vi "Test device info.vi"() -> ()   [LabVIEW 2020, in "XML Handler.lvclass"]
uses:
  XML Handler.lvclass
  Devices/Controls/Device Information Cluster.ctl
  Devices/Controls/Register to Write.ctl
  XML Handler.lvclass/XML Handler.ctl
  <resource>/objmgr/DOMUserDefRef.rc
  Test Framework/Test Framework.lvclass
  Devices/PIC-device/PIC-Device.lvclass
  Devices/Device.lvclass
panel:
  in  "Output File Folder":path
  out "XML":string
  in  "Device Information":T1[](array[typedef])
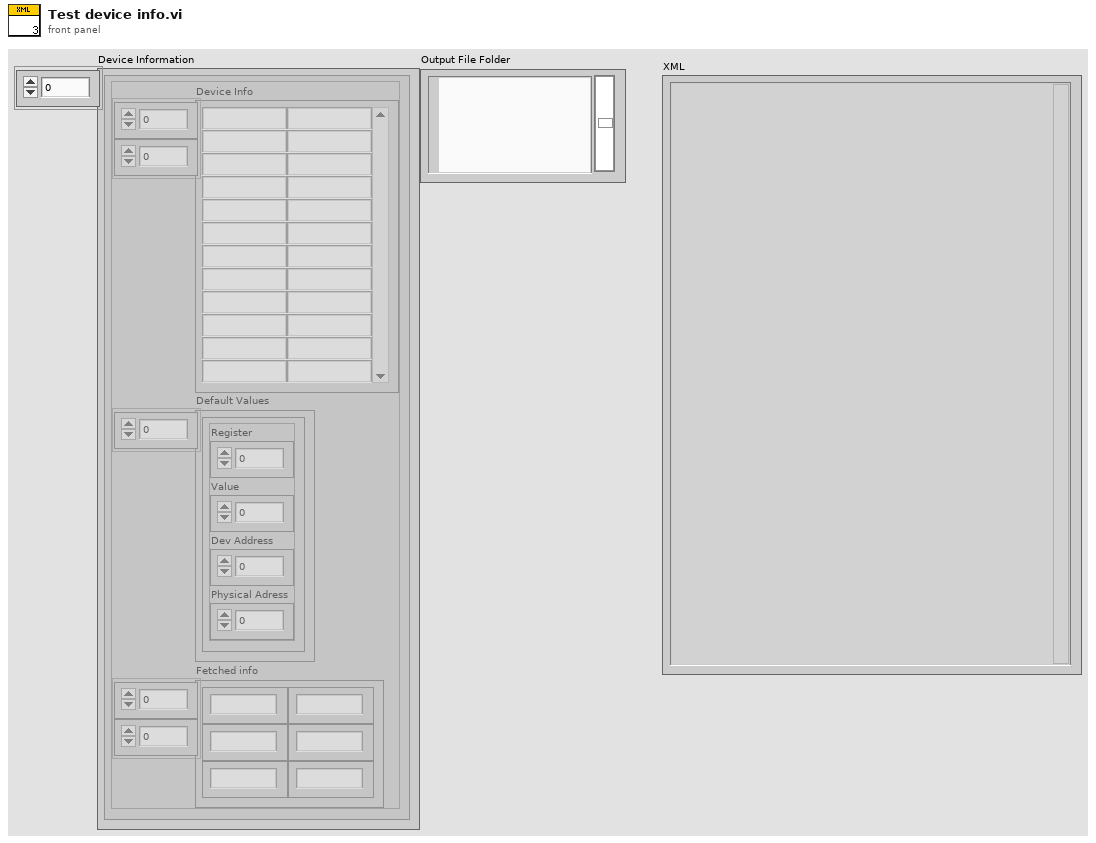
[diagram p1: front panel]
types:
  T1 = typedef "Device.lvclass/Device Information Cluster.ctl" = cluster{"Device Info":string[][], "Default Values":T2[], "Fetched info":string[][]}
  T2 = typedef "PIC-Device.lvclass/Register to Write.ctl" = cluster{"Register":u32, "Value":u32, "Dev Address":u32, "Physical Adress":u32}
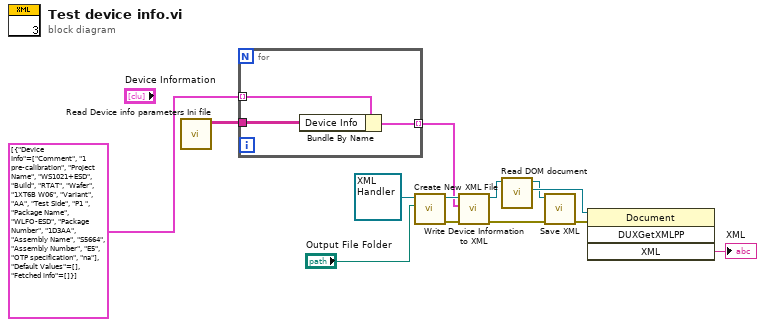
[diagram p0: block diagram]
diagram:
  n1 = call "Read Device info parameters Ini file.vi"() -> ("Instrument info"=w4:string[][])  [unwired: 8 in, 3 out]
  n2 = for {
    tunnel: T1[] [{"Device Info"=[["Comment", "1 pre-calibration"], ["Project Name", "WS1021+ESD"], ["Build", "RTAT"], ["Wafer", "1XT6B W06"], ["Variant", "AA"], ["Test Side", "P1 "], ["Package Name", "WLFO-ESD"], ["Package Number", "1D3AA"], ["Assembly Name", "S5664"], ["Assembly Number", "E5"], ["OTP specification", "na"]], "Default Values"=[], "Fetched info"=[]}] ("Device Info") -> [w16] mode=indexing
    tunnel: w4 -> [w15]
    tunnel: [w14] -> w3 mode=indexing
    n3 = Bundle By Name(cluster=w16, "Device Info"=w15) -> (w14:T1)
  }
  n4 = call "Create New XML File.vi"("Output File Folder"="Output File Folder", "XML Handler in"=refnum<class "XML Handler.lvclass"> refnum) -> ("error out"=w11:errorcluster, "XML Handler out"=w12:refnum<class "XML Handler.lvclass">)  [unwired: 8 in]
  n5 = call "Write Device Information to XML.vi"("error in (no error)"=w11, "Device Information"=w3, "XML Handler in"=w12) -> ("error out"=w5:errorcluster, "XML Handler out"=w10:refnum<class "XML Handler.lvclass">)  [unwired: 7 in]
  n6 = call "Read DOM document.vi"("XML Handler in"=w10) -> ("DOM document"=w9:refnum<k20>, "XML Handler out"=w6:refnum<class "XML Handler.lvclass">)  [unwired: 9 in]
  n7 = call "Save XML.vi"("error in (no error)"=w5, "XML Handler in"=w6) -> ("error out"=w2:errorcluster)  [unwired: 8 in, 1 out]
  n8 = invoke class="Document" method="DUXGetXMLPP"(reference=w9, error in=w2) -> ("XML"=→"XML":string)  [unwired: 2 in, 3 out]
